vi "asap_test.vi"() -> (4 "Channel signal":waveform(dbl)(graph))   [LabVIEW 2014]
uses:
  micron/labview/testing/log_event.ctl
  micron/labview/manipulator/squiggle/Host/i2c_interface.ctl
  micron/labview/manipulator/squiggle/Host/fpga_reference.ctl
  micron/labview/initialization/micron_config.ctl
  micron/labview/testing/Micron params.ctl
  micron/labview/testing/stimulus.ctl
  micron/labview/testing/injection_point.ctl
  micron/labview/filtering/goal_loop_parms.ctl
  micron/labview/testing/mode_conrols.ctl
  micron/labview/testing/manipulator_cal.ctl
  probe_calibration.ctl
  micron/labview/host/network_params.ctl
  micron/labview/cancellation/sq_control_params.ctl
  micron/labview/cancellation/decoupled_gain.ctl
  micron/labview/cancellation/estimation_controls.ctl
  <vilib>/Analysis/2dsp.llb/Real FFT.vi
  initialization/globals.vi
  <vilib>/DAQmx/read.llb/DAQmx Read (Analog 2D DBL NChan NSamp).vi
  <vilib>/express/express analysis/Spectral/Block/exnSpectralBlock spectral measurements PSD poly.vi
  <vilib>/express/express analysis/Spectral/Block/exnSpectralBlock spectral measurements PSD DDT.vi
  <vilib>/express/express analysis/Spectral/XNode/ExpressSpectralMeasurementsBlockNode.xnode
  <vilib>/Analysis/NI_AALPro.lvlib
panel:
  in  "Store gain cal":bool
  out "Carrier frequencies":sgl[][](array[numeric]) format="%#_3p"
  out "Gain calibration":sgl[][](array[numeric]) format="%6.4f"
  in  "Settling delay":i32=10
  in  "Gain calibrate":bool
  in  "Light enable":bool[](array[boolean])=[TRUE, TRUE, TRUE, TRUE, TRUE, TRUE]
  out "Warning":bool
  out "Error":bool
  out "Status":T1[](array[typedef]) {"Timestamp" format="%<%.3X>T"}
  out "Position valid":bool
  out "Channel spectrum":waveform(dbl)(graph)
  in  "Display demodulated":bool
  in  "Restart Averaging":bool
  out "Above 100 Hz":dbl[](array[numeric]) format="%#.2f"
  out "RMS":dbl[](array[numeric]) format="%#.2f"
  out "DC":dbl[](array[numeric]) format="%#.2f"
  in  "Use LUT":bool
  in  "Finder":bool
  in  "Light config":bool[](array[boolean])=[TRUE, TRUE, TRUE, TRUE, TRUE, TRUE]
  out "Output rate (s/s)":dbl
  in  "Updates/sec":sgl=4.0
  in  "stop":bool
  out "max RMS":dbl format="%#_4p"
  out "RMS":dbl[](array[numeric]) format="%#_4p"
  in  "Point selection":T2(ring)
  out "Position Power Spectral Density":dynamicdata(graph) caption="FFT - (RMS)"
  out "Z mismatch":sgl[][](array[numeric]) format="%#.1f"
  out "Sum amplitudes (V)":sgl[][](array[numeric]) format="%#_6f"
  in  "Compensate":bool
  out "Phase errors (degrees)":sgl[][](array[numeric]) format="%6.2f"
  out "max offset":dbl format="%#_4p"
  out "Mean":dbl[](array[numeric]) format="%#7_4p"
  out "max peak":dbl format="%#_4f"
  out "Peak":dbl[](array[numeric]) format="%#_4f"
  in  "Display channel":i32 min=0 max=7
  # "Channel voltages"
  # "Max:"
  # "X"
  # "Z0"
  # "Y"
  # "Z1"
  # "Z mismatch (microns)"
  # "Frequencies"
  # "Position"
  # "3D magnitude:"
  # "Gain calibration requires a special test cable inside the electronics box."
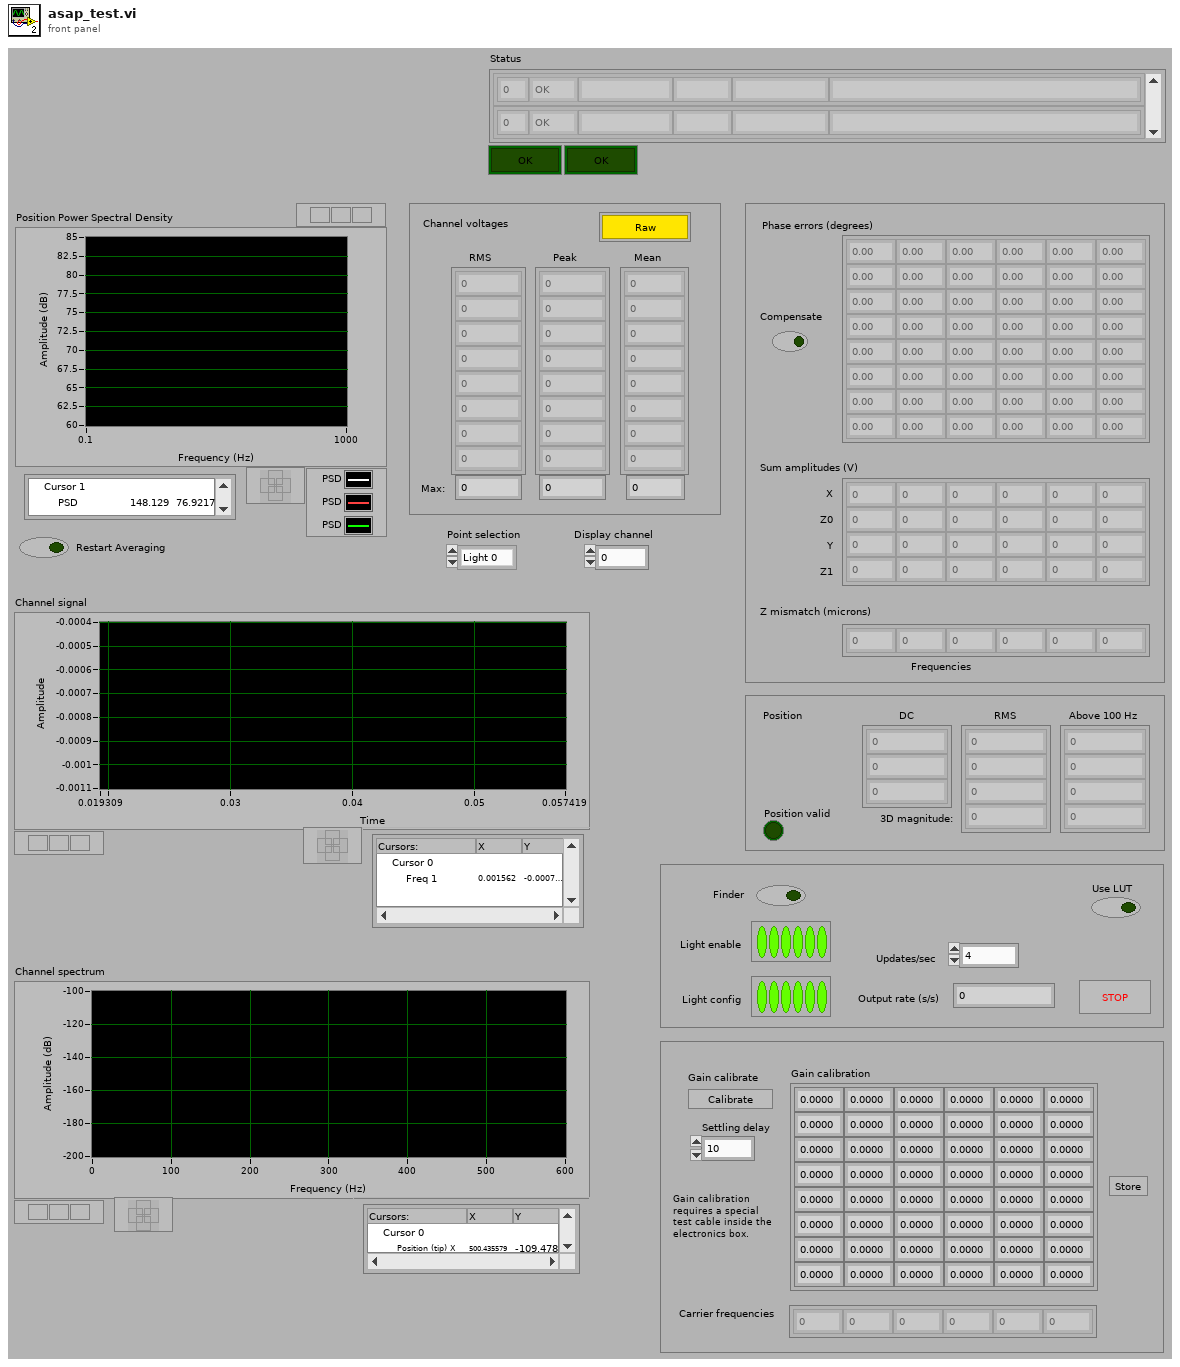
[diagram p1: front panel]
types:
  T1 = typedef "log_event.ctl" = cluster{"Facility ID":i32, "Severity":enum16{"OK", "Debug", "Warn", "Error"}, "Timestamp":timestamp, "Facility":string, "State":string, "Message":string}
  T2 = enum16{"Light 0", "Light 1", "Light 2", "Light 3", "Light 4", "Light 5"}
  T3 = typedef "configuration.ctl" = cluster{"Calibration data":T4, "Block size":i32, "Tasks":cluster{"Analog Input":refnum<k21>, "Counters":refnum<k21>[], "Digital out":refnum<k21>}, "Light enables":bool[]}
  T4 = typedef "asap_calibration.ctl" = cluster{"T1":T5, "K1":T5, "T2":T5, "K2":T5, "Sensor LUT":sgl[][][][]}
  T5 = typedef "NI_Matrix.lvlib/RealMatrix.ctl" = dbl[][]
  T6 = typedef "i2c_interface.ctl" = cluster{"FPGA VI Reference":T7}
  T7 = typedef "fpga_reference.ctl" = refnum<k20>
  T8 = typedef "micron_config.ctl" = cluster{"rt fifo":refnum<k33>, "Analog output task":refnum<k21>, "Analog output task 2":refnum<k21>, "Stimulus AO task":refnum<k21>, "Low-rate AIN task":refnum<k21>, "Pedal out task":refnum<k21>, "Pedal in task":refnum<k21>, "Loop timing source":string, "Relay out task":refnum<k21>, "Send UDP Conn":refnum<k16>, "Recv UDP Conn":refnum<k16>, "Host Addr":u32, "I2C interface":T6, "trace_start notifier":refnum<notifier>, "trace_done notifier":refnum<notifier>, "ASAP FIFO":refnum<k33>}
  T9 = cluster{"averaging mode":u16, "weighting mode":u16, "number of averages":u32}
  T10 = cluster{"dB On (F)":bool, "unwrap phase (F)":bool, "convert to degree (F)":bool}
  T11 = enum16{"ASAP/Trigger", "ASAP/Finder", "ASAP/Micron", "ASAP/Micron 2", "Micron 6DOF"}
  T12 = cluster{"Analog Input":refnum<k21>, "Counters":refnum<k21>[], "Digital out":refnum<k21>}
  T13 = cluster{"seconds since 1Jan1904":timestamp, "Sample interval (sec)":dbl}
  T14 = cluster{"X values":waveform(sgl), "Y values":waveform(sgl), "Z values":waveform(sgl)}[]
  T15 = cluster{"X values":waveform(sgl), "Y values":waveform(sgl), "Z values":waveform(sgl)}
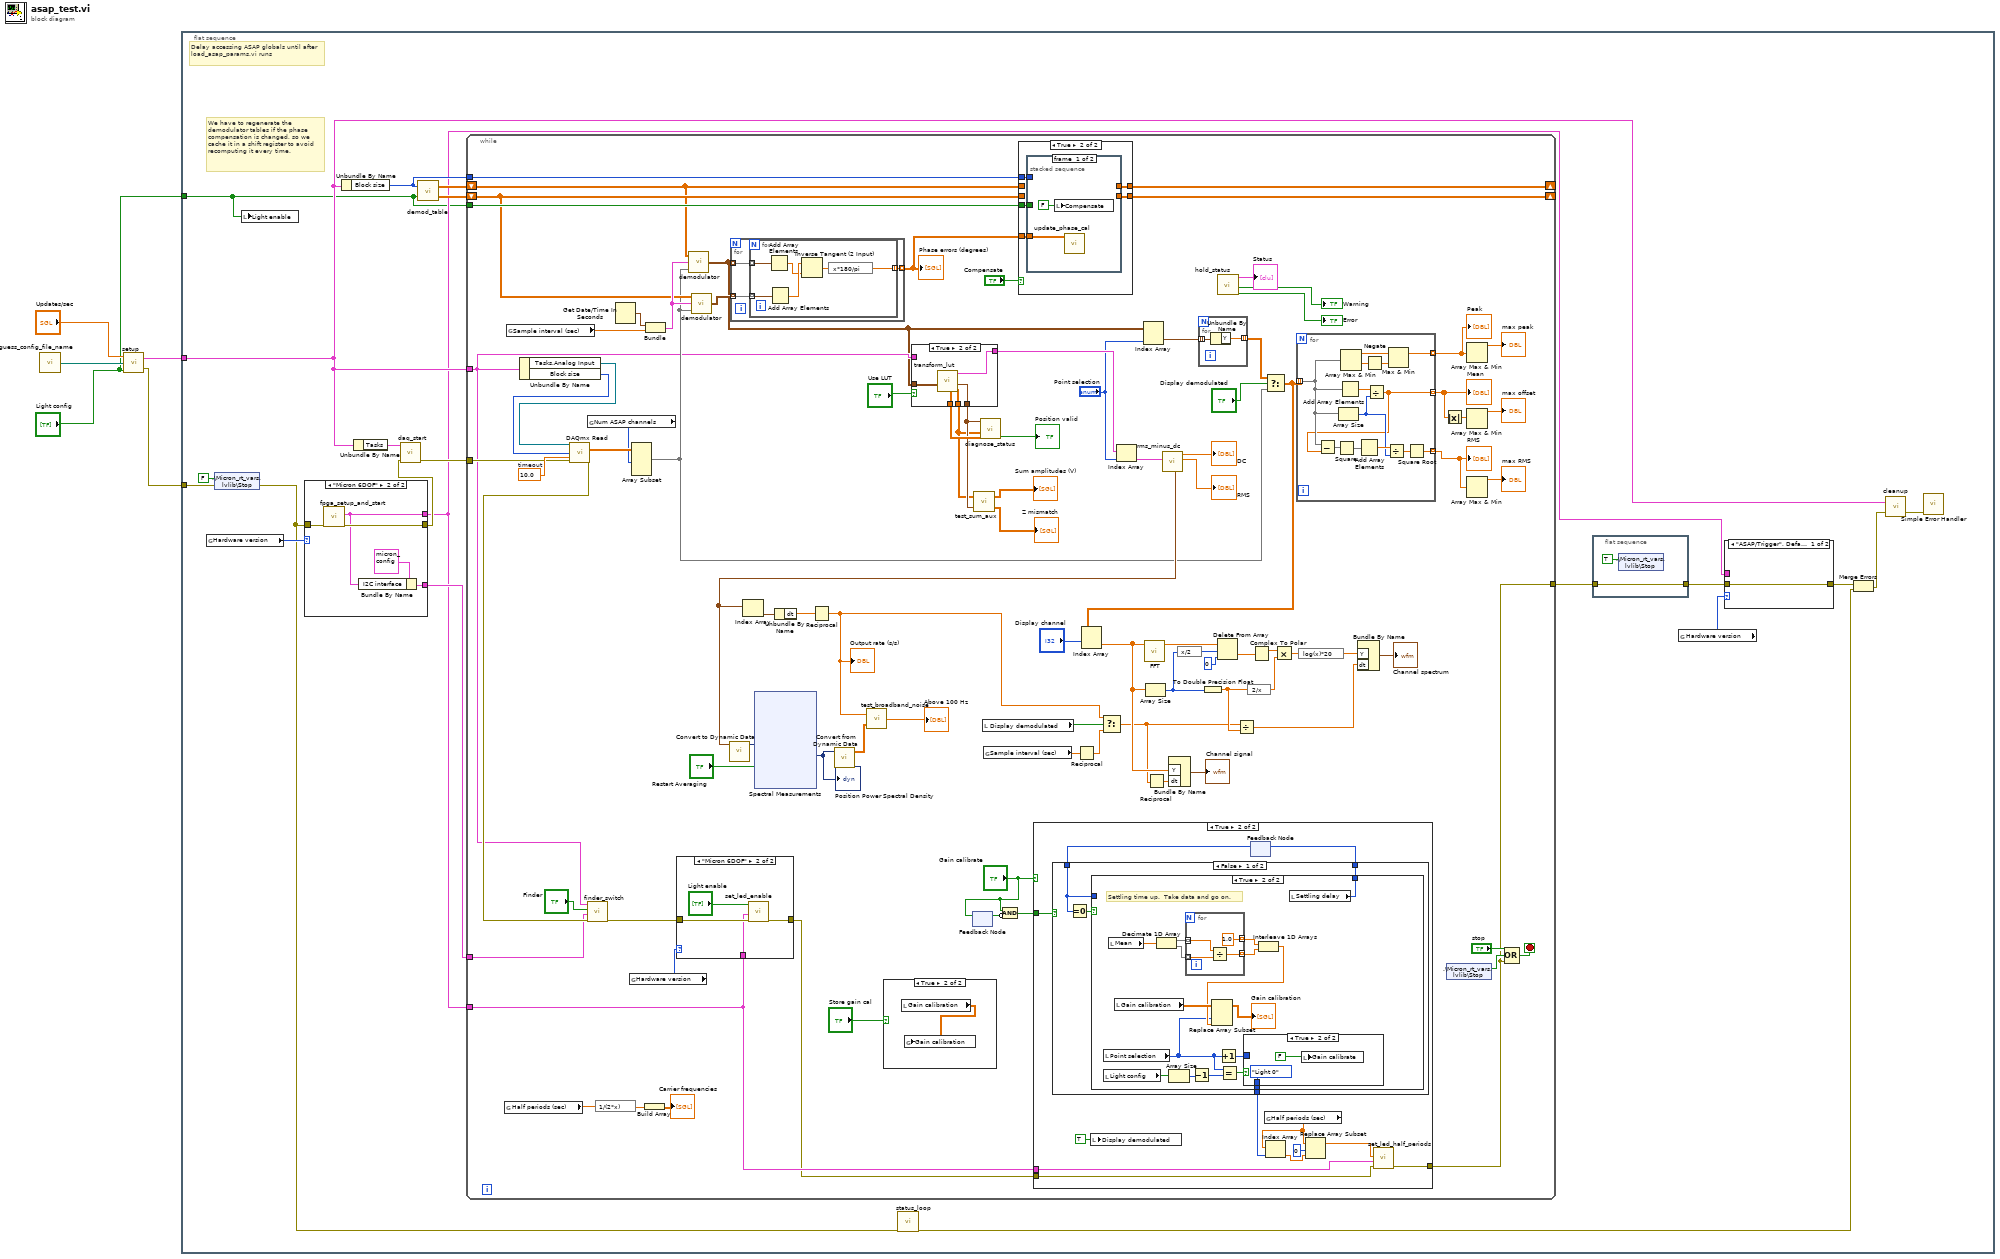
[diagram p0: block diagram]
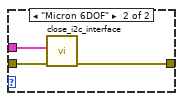
[diagram p2: hidden frame]
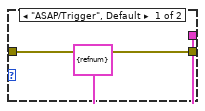
[diagram p3: hidden frame]
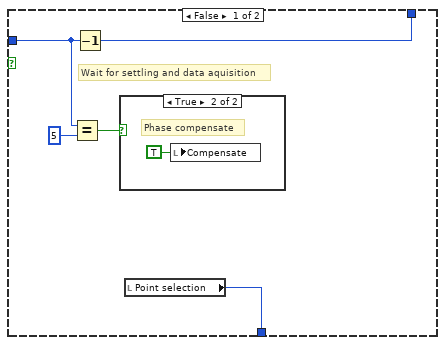
[diagram p6: hidden frame]
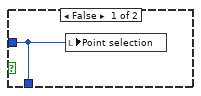
[diagram p8: hidden frame]
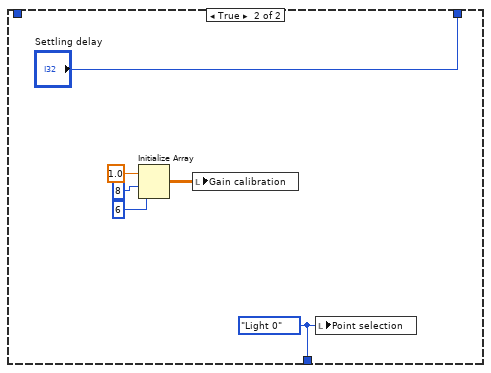
[diagram p9: hidden frame]
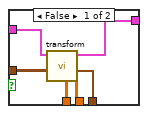
[diagram p11: hidden frame]
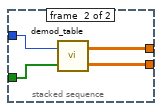
[diagram p13: hidden frame]
diagram:
  n1 = call "guess_config_file_name.vi"() -> ("config file path"=w4:path)
  n2 = call "setup.vi"("Light enables"="Light config", "Calibration file name"=w4, "Updates/sec"="Updates/sec") -> ("error out"=w1:errorcluster, "Configuration"=w3:T3)  [unwired: 1 out]
  n3 = flat-sequence {
    tunnel: w3 -> [w22]
    tunnel: "Light config" -> [w8]
    tunnel: w1 -> [w16]
    frame #0 {
      # "Delay accessing ASAP globals until after load_asap_params.vi runs"
      # "We have to regenerate the demodulator tables if the phase compensation is changed, so we cache it in a shift register to avoid recomputing it every time."
      n4 = global read "globals.vi" "Hardware version"() -> (w19:T11)
      n5 = shared-variable ".\\Micron_rt_vars.lvlib\\Stop"(FALSE ("Stop"), error in=w16) -> (error out=w15:errorcluster)
      n6 = local write "Light enable"(w8) -> ()
      n7 = case shown="\"Micron 6DOF\"" w19 {
        tunnel: w15 -> [w34 w39]
        tunnel: [w34 w38] -> w20
        tunnel: [T6 {"FPGA VI Reference"=refnum} ("I2C interface") w36] -> w9
        tunnel: [_ w35] -> w17
        frame "ASAP/Trigger", Default {
        }
        frame "Micron 6DOF" {
          n8 = call "fpga_setup_and_start.vi"("error in"=w39) -> ("error out"=w38:errorcluster, "I2C interface"=w36:T6)  [unwired: 9 in]
          n9 = Bundle By Name(cluster=T8 {"rt fifo"=refnum, "Analog output task"="", "Analog output task 2"="", "Stimulus AO task"="", "Low-rate AIN task"="", "Pedal out task"="", "Pedal in task"="", "Loop timing source"="", "Relay out task"="", "Send UDP Conn"=refnum, "Recv UDP Conn"=refnum, "Host Addr"=0, "I2C interface"={"FPGA VI Reference"=refnum}, "trace_start notifier"=refnum, "trace_done notifier"=refnum, "ASAP FIFO"=refnum} ("Micron config"), "I2C interface"=w36) -> (w35:T8)
        }
      }
      n10 = Unbundle By Name(w22) -> ("Block size"=w21:i32)
      n11 = Unbundle By Name(w22) -> ("Tasks"=w25:T12)
      n12 = call "daq_start.vi"("error in"=w20, "Tasks"=w25) -> ("error out"=w24:errorcluster)  [unwired: 9 out]
      n13 = call "demod_table.vi"("Light enables"=w8, "Block size"=w21) -> ("Cosine table"=w23:dbl[][][], "Sine table"=w10:dbl[][][])
      n14 = while {
        tunnel: w22 -> [w53]
        tunnel: w24 -> [w110]
        shift-right: [w108] -> _
        shift-left: w10 -> [w104]
        shift-right: [w109] -> _
        shift-left: w23 -> [w105]
        tunnel: w21 -> [w107]
        tunnel: w8 -> [w106]
        tunnel: w17 -> [w59]
        tunnel: w9 -> [w46]
        tunnel: [w44] -> w7
        stop <- w130 stop-if-true
        w133 = 10.0  # timeout
        n15 = global read "globals.vi" "Half periods (sec)"() -> (w43:dbl[])
        n16 = global read "globals.vi" "Sample interval (sec)"() -> (w112:dbl)
        n17 = Unbundle By Name(w53) -> ("Tasks.Analog Input"=w132:refnum<k21>, "Block size"=w128:i32)
        n18 = call-poly <vilib>:"DAQmx Read.vi"("task/channels in"=w132, "number of samples per channel"=w128, "timeout"=w133, "error in"=w110) -> ("data"=w115:dbl[][], "error out"=w96:errorcluster)  [unwired: 10 out]
        n19 = global read "globals.vi" "Num ASAP channels"() -> (w114:i32)
        n20 = call "finder_switch.vi"("error in"=w96, "Micron config"=w59, "Finder"="Finder", "Configuration"=w53) -> ("error out"=w51:errorcluster)  [unwired: 5 out]
        n21 = expression code="1/(2*x)"(w43) -> (w42:dbl[])
        n22 = Get Date/Time In Seconds() -> (seconds since 1Jan1904=w113:timestamp)
        n23 = global read "globals.vi" "Hardware version"() -> (w50:T11)
        n24 = Array Subset(array=w115, length (row)=w114) -> (w87:dbl[][])  [unwired: 3 in]
        n25 = Build Array(w42) -> (→"Carrier frequencies":dbl[][])
        n26 = Bundle("seconds since 1Jan1904"=w113, "Sample interval (sec)"=w112) -> (w111:T13)  [unwired: 1 out]
        n27 = case shown="\"Micron 6DOF\"" w50 {
          tunnel: w51 -> [w187 w191]
          tunnel: [w187 w190] -> w45
          tunnel: w46 -> [_ w189]
          frame "ASAP/Trigger", Default {
          }
          frame "Micron 6DOF" {
            n28 = call "set_led_enable.vi"("error in"=w191, "I2C interface"=w189, "LED enables"="Light enable") -> ("error out"=w190:errorcluster)  [unwired: 8 in]
          }
        }
        n29 = call "demodulator.vi"("ADC data"=w87, "timestamp"=w111, "Demodulator table"=w104) -> ("Demodulated signals"=w52:waveform(sgl)[][])
        n30 = call "demodulator.vi"("ADC data"=w87, "timestamp"=w111, "Demodulator table"=w105) -> ("Demodulated signals"=w120:waveform(sgl)[][])
        n31 = for {
          tunnel: w52 -> [w243] mode=indexing
          tunnel: w120 -> [w242] mode=indexing
          tunnel: [w241] -> w91 mode=indexing
          n32 = for {
            tunnel: w243 -> [w249] mode=indexing
            tunnel: w242 -> [w248] mode=indexing
            tunnel: [w247] -> w241 mode=indexing
            n33 = Add Array Elements(numeric array=w249) -> (sum=w244:sgl)
            n34 = Add Array Elements(numeric array=w248) -> (sum=w245:sgl)
            n35 = Inverse Tangent (2 Input)(1:w244, 2:w245) -> (0:w246:sgl)
            n36 = expression code="x*180/pi"(w246) -> (w247:sgl)
          }
        }
        "Phase errors (degrees)" <- w91
        n37 = case shown="True" "Store gain cal" {
          frame False {
          }
          frame True {
            n38 = local read "Gain calibration"() -> (w134:sgl[][])
            n39 = global write "globals.vi" "Gain calibration"(w134) -> ()
          }
        }
        n40 = case shown="True" "Use LUT" {
          tunnel: w52 -> [w209 w214]
          tunnel: [w208 w210] -> w98
          tunnel: [w207 w213] -> w119
          tunnel: [w206 w212] -> w117
          tunnel: w53 -> [w205 _]
          tunnel: [w204 w211] -> w92
          frame False {
            n41 = call "transform.vi"("Demodulated signals"=w209, "Configuration"=w205) -> ("Sum amplitudes"=w208:sgl[][], "Match error"=w206:waveform(sgl)[], "XYZ out"=w204:T14, "Axis positions"=w207:sgl[][])  [unwired: 6 out]
          }
          frame True {
            n42 = call "transform_lut.vi"("Demodulated signals"=w214) -> ("Sum amplitudes"=w210:sgl[][], "Match error"=w212:waveform(sgl)[], "XYZ out"=w211:T14, "Axis positions"=w213:sgl[][])  [unwired: 1 in, 6 out]
          }
        }
        n43 = feedback-in #1("Gain calibrate") -> ()
        n44 = feedback #1() -> (w49:bool)  [unwired: 1 in]
        n45 = call "test_sum_aux.vi"("Z mismatch"=w117, "Sum amplitudes"=w98) -> ("Real 2D Array"=→"Z mismatch":sgl[][], "Array"=→"Sum amplitudes (V)":sgl[][])
        n46 = call "diagnose_status.vi"("Axis positions"=w119, "Sum amplitudes"=w98, "Match error"=w117) -> ("Position valid"=→"Position valid":bool)  [unwired: 8 in]
        n47 = local read "Display demodulated"() -> (w76:bool)
        n48 = global read "globals.vi" "Sample interval (sec)"() -> (w74:dbl)
        n49 = Compound Arithmetic op=AND("Gain calibrate", invert w49) -> (w47:bool)
        n50 = case shown="True" "Compensate" {
          tunnel: [w229 w234] -> w109
          tunnel: [w228 w233] -> w108
          tunnel: w107 -> [_ w232]
          tunnel: w106 -> [_ w231]
          tunnel: w105 -> [w229 _]
          tunnel: w104 -> [w228 _]
          tunnel: w91 -> [_ w230]
          frame False {
          }
          frame True {
            n51 = stacked-sequence {
              tunnel: [_ w240] -> w234
              tunnel: [_ w239] -> w233
              tunnel: w232 -> [_ w238]
              tunnel: w231 -> [_ w237]
              tunnel: w230 -> [w236 _]
              frame #0 {
                n52 = local write "Compensate"(FALSE ("Compensate")) -> ()
                n53 = call "update_phase_cal.vi"("Phase errors"=w236) -> ()  [unwired: 11 in]
              }
              frame #1 {
                n54 = call "demod_table.vi"("Light enables"=w237, "Block size"=w238) -> ("Cosine table"=w240:dbl[][][], "Sine table"=w239:dbl[][][])
              }
            }
          }
        }
        n55 = case shown="True" "Gain calibrate" {
          tunnel: w47 -> [_ w147]
          tunnel: w46 -> [_ w143]
          tunnel: w45 -> [w135 w142]
          tunnel: [w135 w141] -> w44
          frame False {
          }
          frame True {
            n56 = local write "Display demodulated"(TRUE ("Display demodulated")) -> ()
            n57 = feedback #2() -> (w144:i32)  [unwired: 1 in]
            n58 = case shown="False" w147 {
              tunnel: [w150 "Settling delay"] -> w145
              tunnel: w144 -> [w149 _]
              tunnel: [w148 w185] -> w138
              frame False {
                n59 = Equal To 0?(x=w149) -> (x = 0?=w151:bool)
                n60 = case shown="True" w151 {
                  tunnel: [w156 w163] -> w150
                  tunnel: w149 -> [w154 _]
                  tunnel: [w155 w162] -> w148
                  frame False {
                    # "Wait for settling and data aquisition"
                    n61 = Equal?(x=w154, y=5) -> (x = y?=w152:bool)
                    n62 = Decrement(x=w154) -> (x-1=w156:i32)
                    n63 = case shown="True" w152 {
                      frame False {
                      }
                      frame True {
                        # "Phase compensate"
                        n64 = local write "Compensate"(TRUE ("Compensate")) -> ()
                      }
                    }
                    n65 = local read "Point selection"() -> (w155:T2)
                  }
                  frame True {
                    # "Settling time up.  Take data and go on."
                    n66 = local read "Point selection"() -> (w159:T2)
                    n67 = local read "Light config"() -> (w166:bool[])
                    n68 = local read "Mean"() -> (w158:dbl[])
                    n69 = local read "Gain calibration"() -> (w169:sgl[][])
                    n70 = Decimate 1D Array(w158) -> (w173:dbl[], w172:dbl[])
                    n71 = Array Size(array=w166) -> (size(s)=w161:i32)
                    n72 = for {
                      tunnel: w173 -> [w179] mode=indexing
                      tunnel: w172 -> [w180] mode=indexing
                      tunnel: [w178] -> w170 mode=indexing
                      tunnel: [1.0] -> w171 mode=indexing
                      n73 = Divide(x=w179, y=w180) -> (x/y=w178:dbl)
                    }
                    n74 = Decrement(x=w161) -> (x-1=w160:i32)
                    n75 = Increment(x=w159) -> (x+1=w164:T2)
                    n76 = Equal?(x=w159, y=w160) -> (x = y?=w165:bool)
                    n77 = case shown="True" w165 {
                      tunnel: w164 -> [w174 _]
                      tunnel: [w174 T2."Light 0"] -> w162
                      frame False {
                        n78 = local write "Point selection"(w174) -> ()
                      }
                      frame True {
                        n79 = local write "Gain calibrate"(FALSE ("Amplitude calibrate")) -> ()
                      }
                    }
                    n80 = Interleave 1D Arrays(w171, w170) -> (w168:dbl[])
                    n81 = Replace Array Subset(array=w169, new element=w168, index (col)=w159) -> (→"Gain calibration":sgl[][])  [unwired: 1 in]
                    n82 = local read "Settling delay"() -> (w163:i32)
                  }
                }
              }
              frame True {
                w185 = T2."Light 0" ("Point selection")
                n83 = Initialize Array(sgl 1.0, 8 ("dimension size"), 6 ("dimension size")) -> (w184:sgl[][])
                n84 = local write "Gain calibration"(w184) -> ()
                n85 = local write "Point selection"(w185) -> ()
              }
            }
            n86 = feedback-in #2(w145) -> ()
            n87 = global read "globals.vi" "Half periods (sec)"() -> (w139:dbl[])
            n88 = Index Array(array=w139, index=w138) -> (element=w137:dbl)
            n89 = Replace Array Subset(array=w139, new element=w137, index=0) -> (w136:dbl[])
            n90 = call "set_led_half_periods.vi"("error in"=w142, "I2C interface"=w143, "Half periods (sec)"=w136) -> ("error out"=w141:errorcluster)  [unwired: 8 in]
          }
        }
        n91 = Reciprocal(x=w74) -> (1/x=w73:dbl)
        n92 = Index Array(array=w92, index="Point selection") -> (element=w118:T15)
        n93 = Index Array(array=w52, index (col)="Point selection") -> (element=w86:waveform(sgl)[])  [unwired: 1 in]
        n94 = call "rms_minus_dc.vi"("Signal"=w118) -> ("RMS"=→"RMS":dbl[], "DC"=→"DC":dbl[], "AC signal"=w116:waveform(sgl)[])  [unwired: 8 out]
        n95 = call "Convert to Dynamic Data"("Array of Waveforms"=w116) -> ("Dynamic Data Type"=w97:dynamicdata)  [unwired: 3 out]
        n96 = Index Array(array=w116) -> (element=w77:waveform(sgl))  [unwired: 1 in]
        n97 = xnode "Spectral Measurements"("Signals"=w97, "Restart Averaging"="Restart Averaging") -> ("PSD"=w95:dynamicdata)  [unwired: 1 in, 2 out]
        "Position Power Spectral Density" <- w95
        n98 = Unbundle By Name(w77) -> ("dt"=w78:dbl)
        n99 = Reciprocal(x=w78) -> (1/x=w75:dbl)
        "Output rate (s/s)" <- w75
        n100 = call "Convert from Dynamic Data"("Dynamic Data Type"=w95) -> ("Array"=w94:dbl[][])  [unwired: 3 out]
        n101 = call "test_broadband_noise.vi"("PSD"=w94, "Sample Rate"=w75) -> ("HF amplitude"=→"Above 100 Hz":dbl[])
        n102 = Select(t=w75, s=w76, f=w73) -> (s? t:f=w62:dbl)
        n103 = Reciprocal(x=w62) -> (1/x=w63:dbl)
        n104 = for {
          tunnel: w86 -> [w193] mode=indexing
          tunnel: [w192] -> w85 mode=indexing
          n105 = Unbundle By Name(w193) -> ("Y"=w192:sgl[])
        }
        n106 = call "hold_status.vi"() -> ("Error"=→"Error":bool, "Warning"=→"Warning":bool, "Hold status"=→"Status":T1[])  [unwired: 9 in]
        n107 = Select(t=w85, s="Display demodulated", f=w87) -> (s? t:f=w84:dbl[][])
        n108 = Index Array(array=w84, index (row)="Display channel") -> (element=w65:dbl[])  [unwired: 1 in]
        n109 = call-poly <vilib>:"FFT.vi"("X"=w65) -> ("FFT {X}"=w71:cdb[])  [unwired: 9 in, 1 out]
        n110 = Array Size(array=w65) -> (size(s)=w69:i32)
        n111 = Bundle By Name("Y"=w65, "dt"=w63) -> (→"Channel signal":waveform(dbl))  [unwired: 1 in]
        n112 = expression code="x/2"(w69) -> (w70:i32)
        n113 = To Double Precision Float(number=w69) -> (double precision float=w72:dbl)
        n114 = Delete From Array(array=w71, length=w70, index=0) -> (deleted portion=w68:cdb[])  [unwired: 1 out]
        n115 = Divide(x=w62, y=w72) -> (x/y=w67:dbl)
        n116 = expression code="2/x" ("degrees to radians")(w72) -> (w83:dbl)
        n117 = Complex To Polar(r * e^(i*theta)=w68) -> (r=w82:dbl[])  [unwired: 1 out]
        n118 = Multiply(x=w82, y=w83) -> (x*y=w81:dbl[])
        n119 = for {
          tunnel: w84 -> [w221] mode=indexing
          tunnel: [w224] -> w127 mode=indexing
          tunnel: [w215] -> w100 mode=indexing
          tunnel: [w216] -> w102 mode=indexing
          n120 = Array Size(array=w221) -> (size(s)=w218:i32)
          n121 = Add Array Elements(numeric array=w221) -> (sum=w223:dbl)
          n122 = Array Max & Min(array=w221) -> (max value=w226:dbl, min value=w225:dbl)  [unwired: 2 out]
          n123 = Negate(x=w225) -> (-x=w227:dbl)
          n124 = Divide(x=w223, y=w218) -> (x/y=w215:dbl)
          n125 = Subtract(x=w221, y=w215) -> (x-y=w222:dbl[])
          n126 = Square(x=w222) -> (x^2=w220:dbl[])
          n127 = Add Array Elements(numeric array=w220) -> (sum=w219:dbl)
          n128 = Divide(x=w219, y=w218) -> (x/y=w217:dbl)
          n129 = Max & Min(x=w226, y=w227) -> (max(x,y)=w224:dbl)  [unwired: 1 out]
          n130 = Square Root(x=w217) -> (sqrt(x)=w216:dbl)
        }
        "Peak" <- w127
        "Mean" <- w100
        "RMS" <- w102
        n131 = expression code="log(x)*20"(w81) -> (w80:dbl[])
        n132 = Bundle By Name("Y"=w80, "dt"=w67) -> (→"Channel spectrum":waveform(dbl))  [unwired: 1 in]
        n133 = Absolute Value(x=w100) -> (abs(x)=w101:dbl[])
        n134 = shared-variable ".\\Micron_rt_vars.lvlib\\Stop"() -> (w54:bool)  [unwired: 2 out]
        n135 = Array Max & Min(array=w127) -> (max value=→"max peak":dbl)  [unwired: 3 out]
        n136 = Array Max & Min(array=w101) -> (max value=→"max offset":dbl)  [unwired: 3 out]
        n137 = Array Max & Min(array=w102) -> (max value=→"max RMS":dbl)  [unwired: 3 out]
        n138 = Compound Arithmetic op=OR("stop", w54, w44) -> (w130:bool)
      }
      n139 = call "status_loop.vi"("error in (no error)"=w15) -> ("error out"=w11:errorcluster)  [unwired: 10 in]
      n140 = flat-sequence {
        tunnel: w7 -> [w27]
        tunnel: [w27] -> w6
        frame #0 {
          n141 = shared-variable ".\\Micron_rt_vars.lvlib\\Stop"(TRUE ("Stop")) -> ()  [unwired: 2 out]
        }
      }
      n142 = global read "globals.vi" "Hardware version"() -> (w18:T11)
      n143 = case shown="\"ASAP/Trigger\", Default" w18 {
        tunnel: [w29 w32] -> w13
        tunnel: w9 -> [_ w31]
        tunnel: w6 -> [w29 w30]
        frame "ASAP/Trigger", Default {
        }
        frame "Micron 6DOF" {
          n144 = call "close_i2c_interface.vi"("error in"=w30, "I2C interface"=w31) -> ("error out"=w32:errorcluster)  [unwired: 9 in]
        }
      }
      n145 = Merge Errors(w13, w11) -> (w12:errorcluster)
      n146 = call "cleanup.vi"("error in"=w12, "Configuration"=w22) -> ("error out"=w26:errorcluster)  [unwired: 1 out]
      n147 = call <vilib>:"Simple Error Handler.vi"("error in (no error)"=w26) -> ()  [unwired: 1 in, 8 out]
    }
  }
